vi "SimpleLiveAppProgrammableScanMode.vi"() -> ()   [LabVIEW 2020]
uses:
  C:/Users/Public/Documents/Photometrics/PMQI-LabViewSamples/Examples/2018/Dependencies/PVCamNET.dll
  Dependencies/PVCamNET.dll
panel:
  out "Exp. out":i32
  in  "Trigger Out Behaviour":string(combo)
  out "Boolean":bool
  in  "Scan Direction Reset":bool
  out "Scan Line Time":dbl format="%#_14g"
  in  "Scan Width":dbl
  in  "Scan Line Delay":dbl
  in  "Scan Direction":string(combo)
  in  "Scan Mode":string(combo)
  in  "Exposure Time":dbl
  in  "Live":bool
  in  "Camera Status":bool
  in  "Uninit":bool
  in  "Live stop":bool
  in  "Live start":bool
  in  "Open":bool
  # "SimpleLiveAppProgrammableScanMode.vi\n\nDescription:\nThis sample code lets the user use programmable scan\n mode in an event driven structure.\n\nSteps to run:\n1. Click \"Run\"\n2. Click \"Open\"\n3. Enter Exposure Time\n4. Select Scan Mode. \n5. Set Scan Line Delay or Scan Width\n6. Select Scan Direction\n7. Click \"Live start\"\n8. Click \"Live stop\"\n9. Click \"Close\""
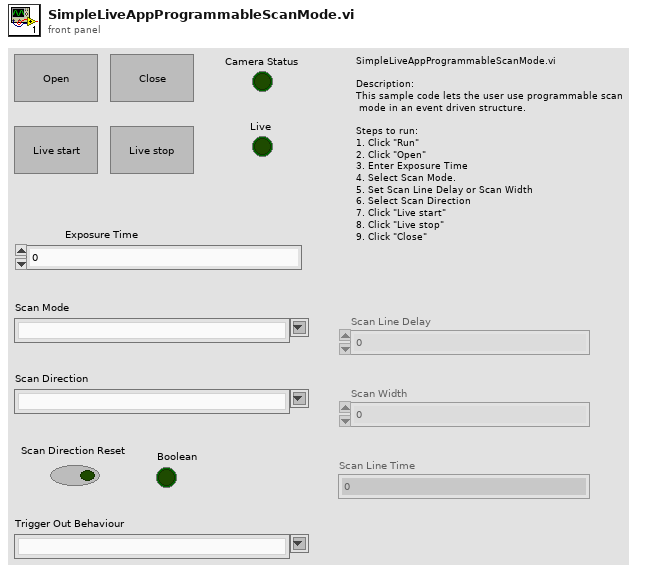
[diagram p1: front panel]
types:
  T1 = enum8{"Enabled", "Disabled", "Disabled and Grayed Out"}
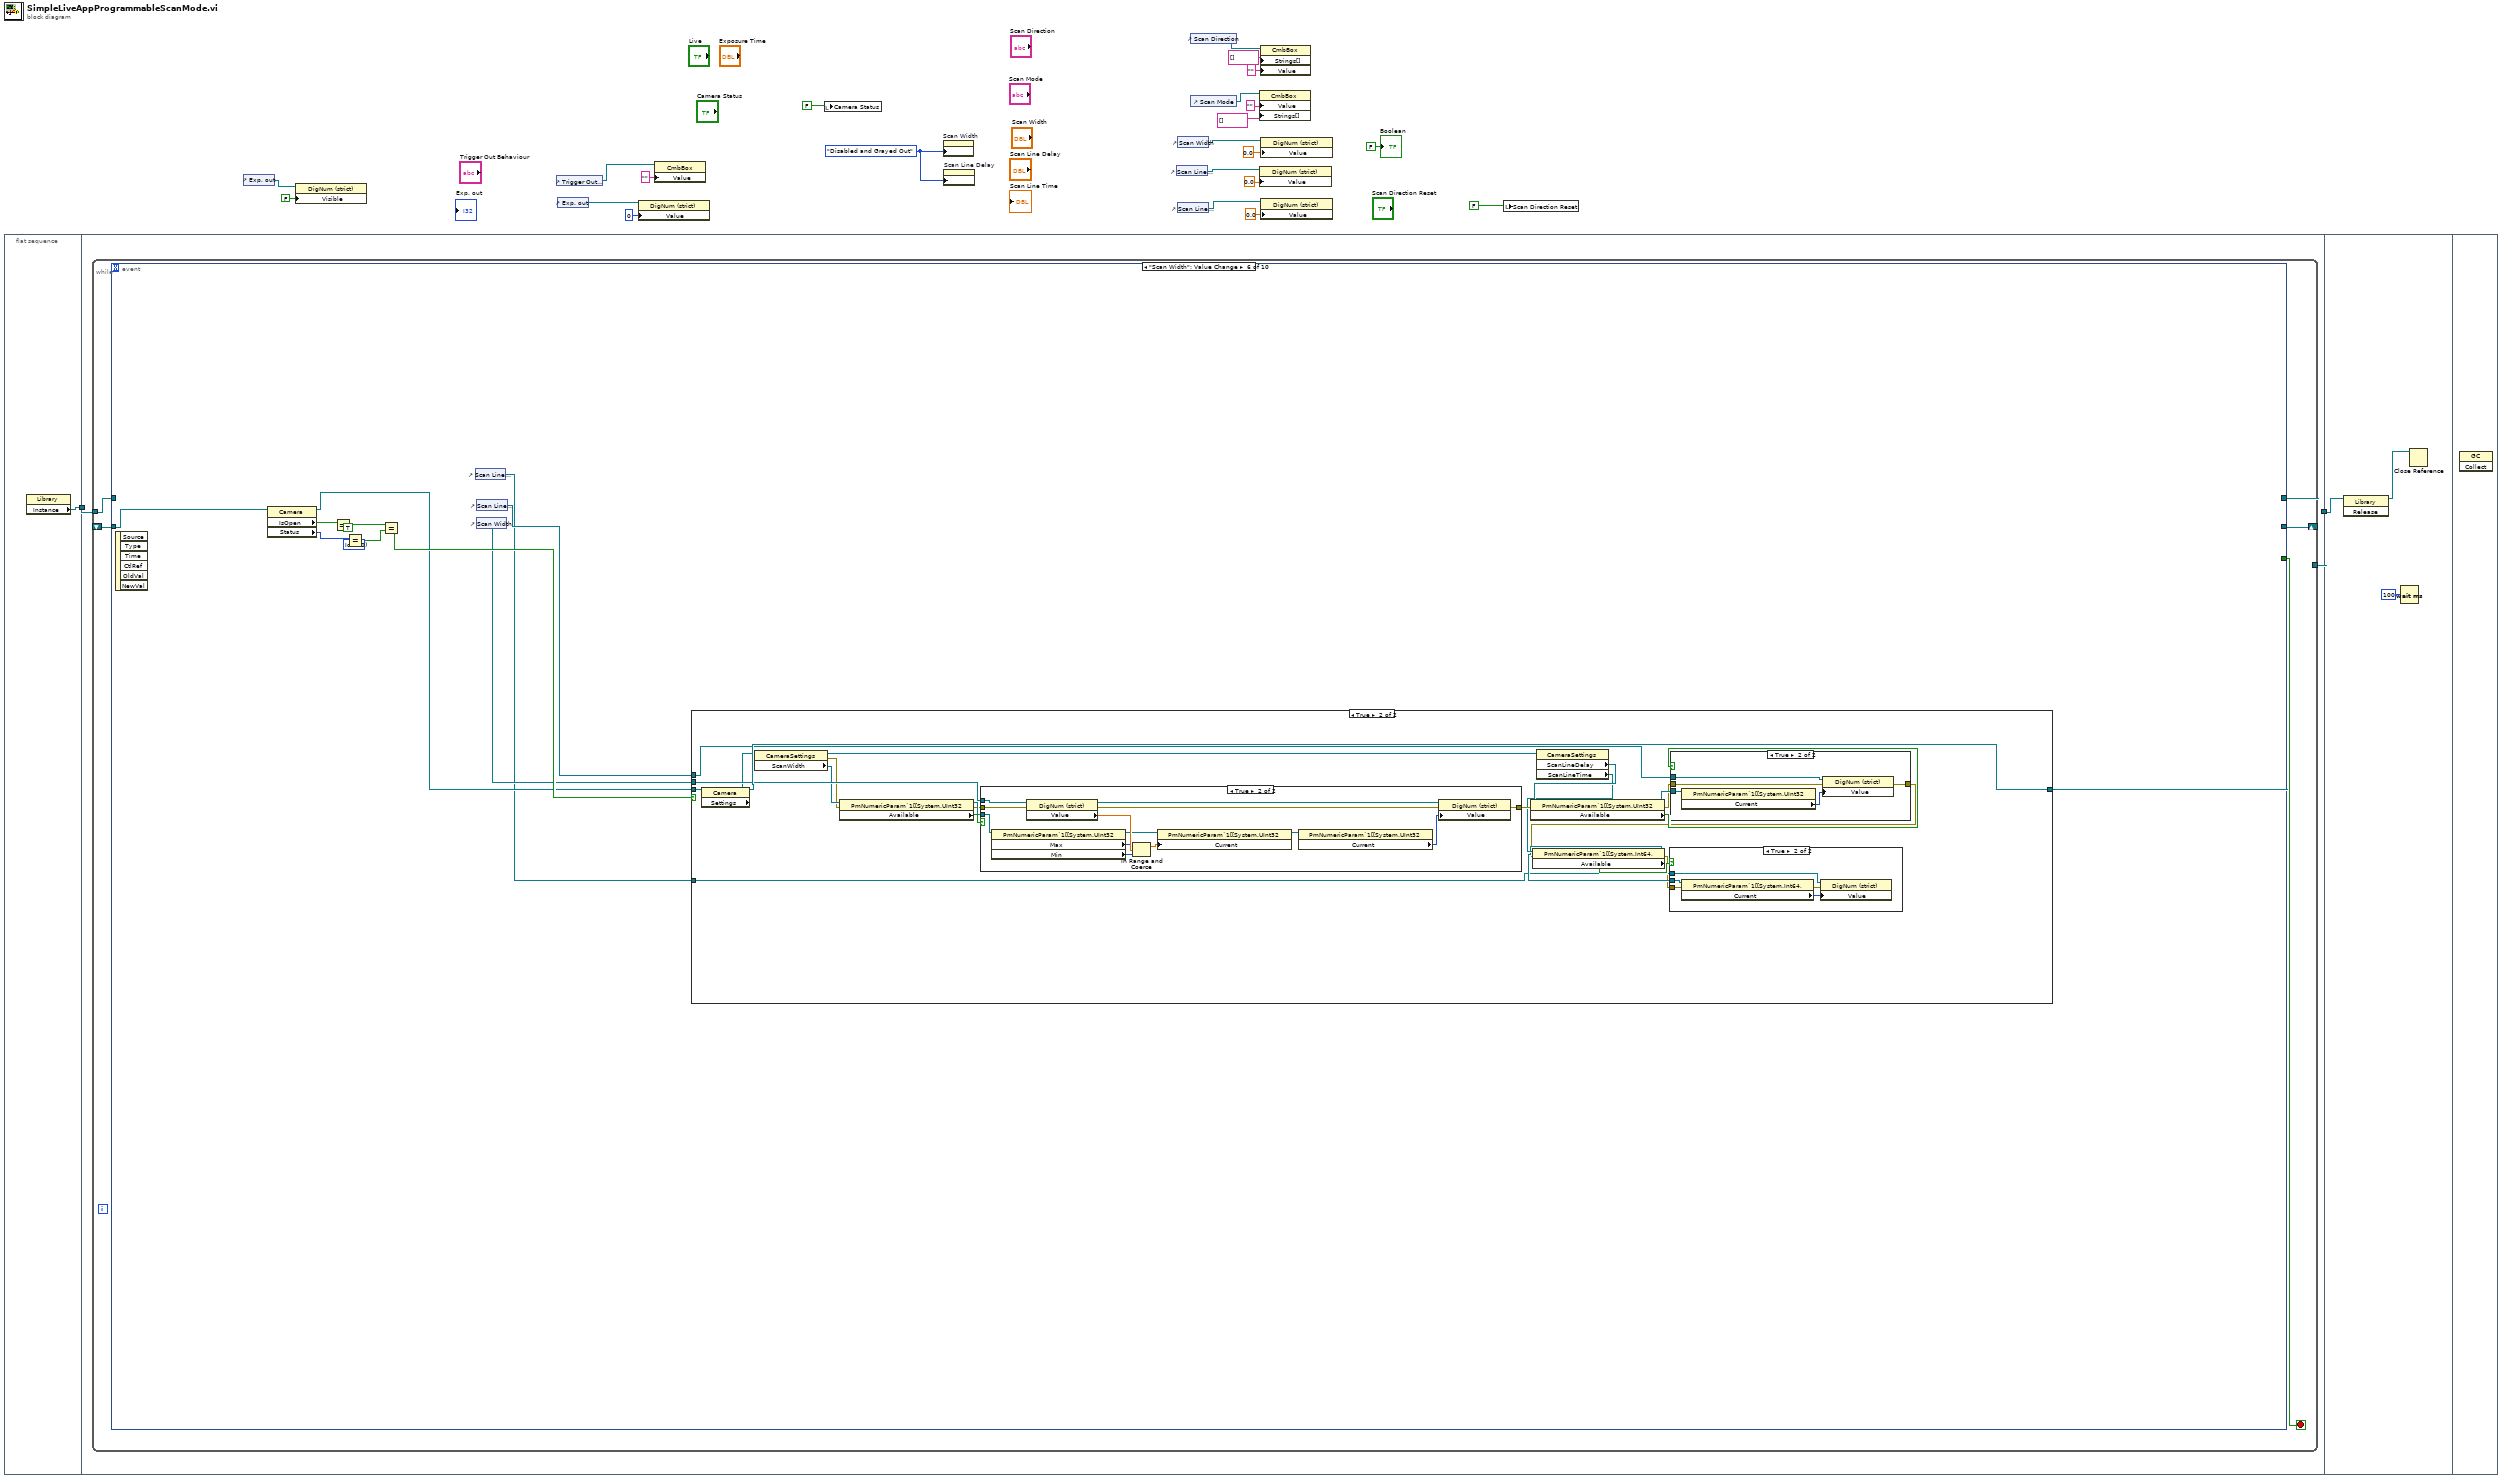
[diagram p0: block diagram]
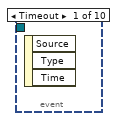
[diagram p2: hidden frame]
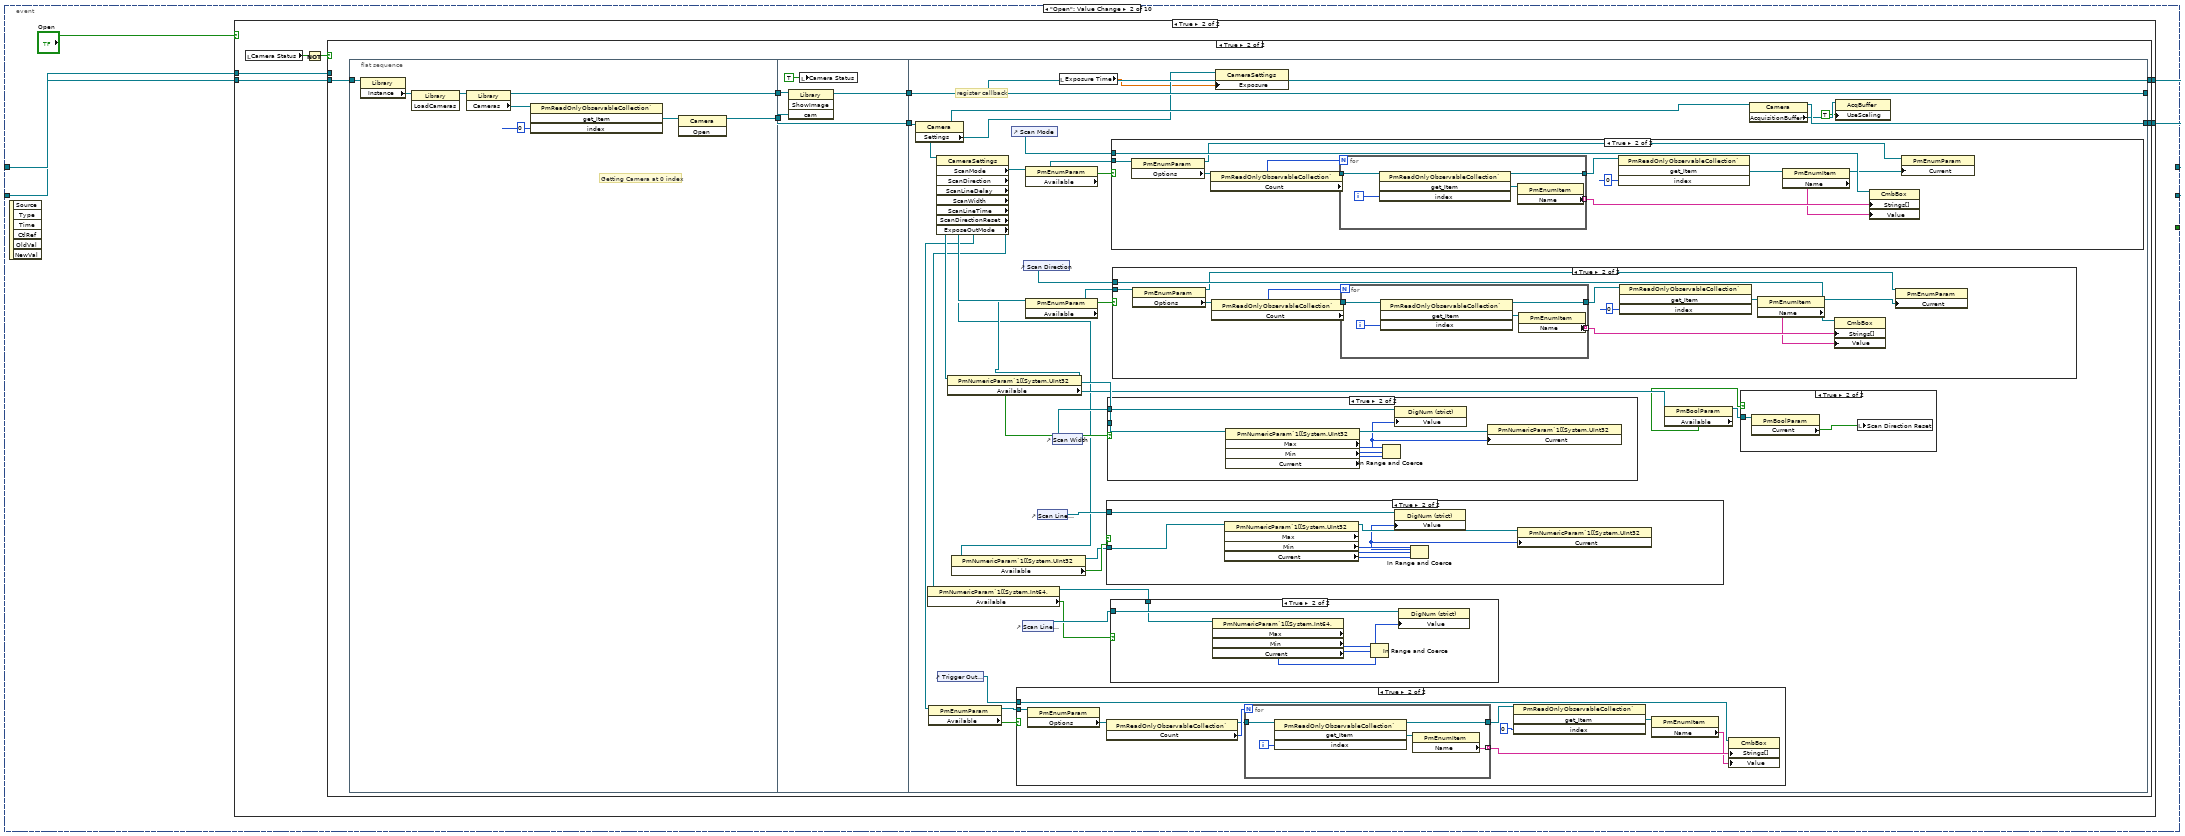
[diagram p3: hidden frame]
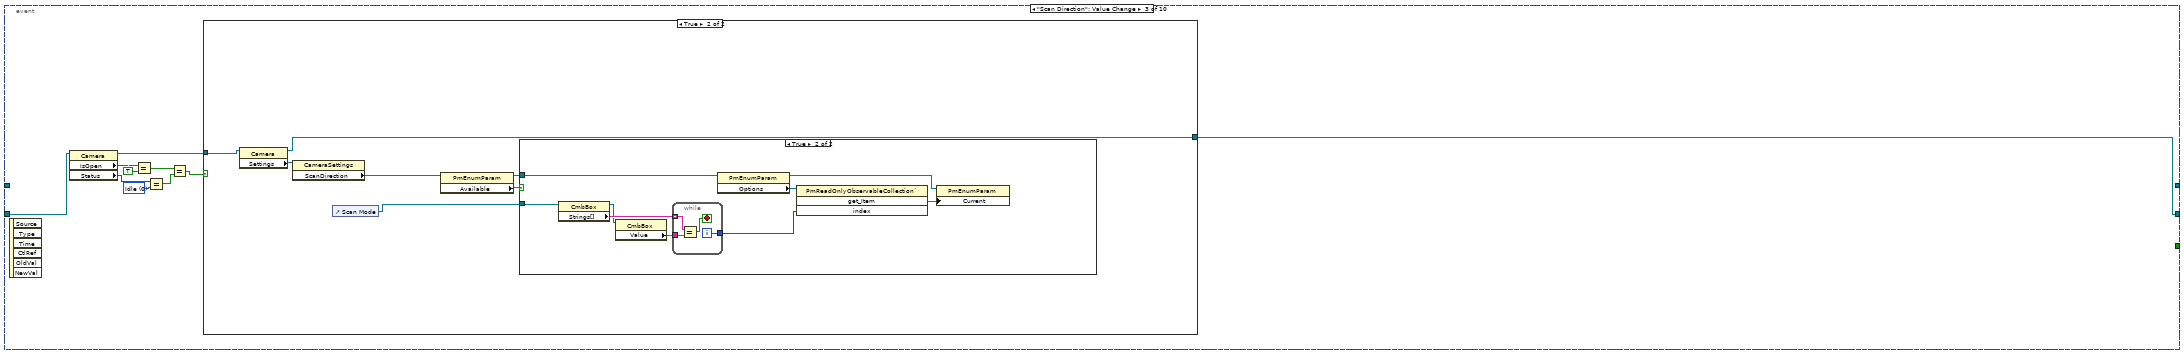
[diagram p13: hidden frame]
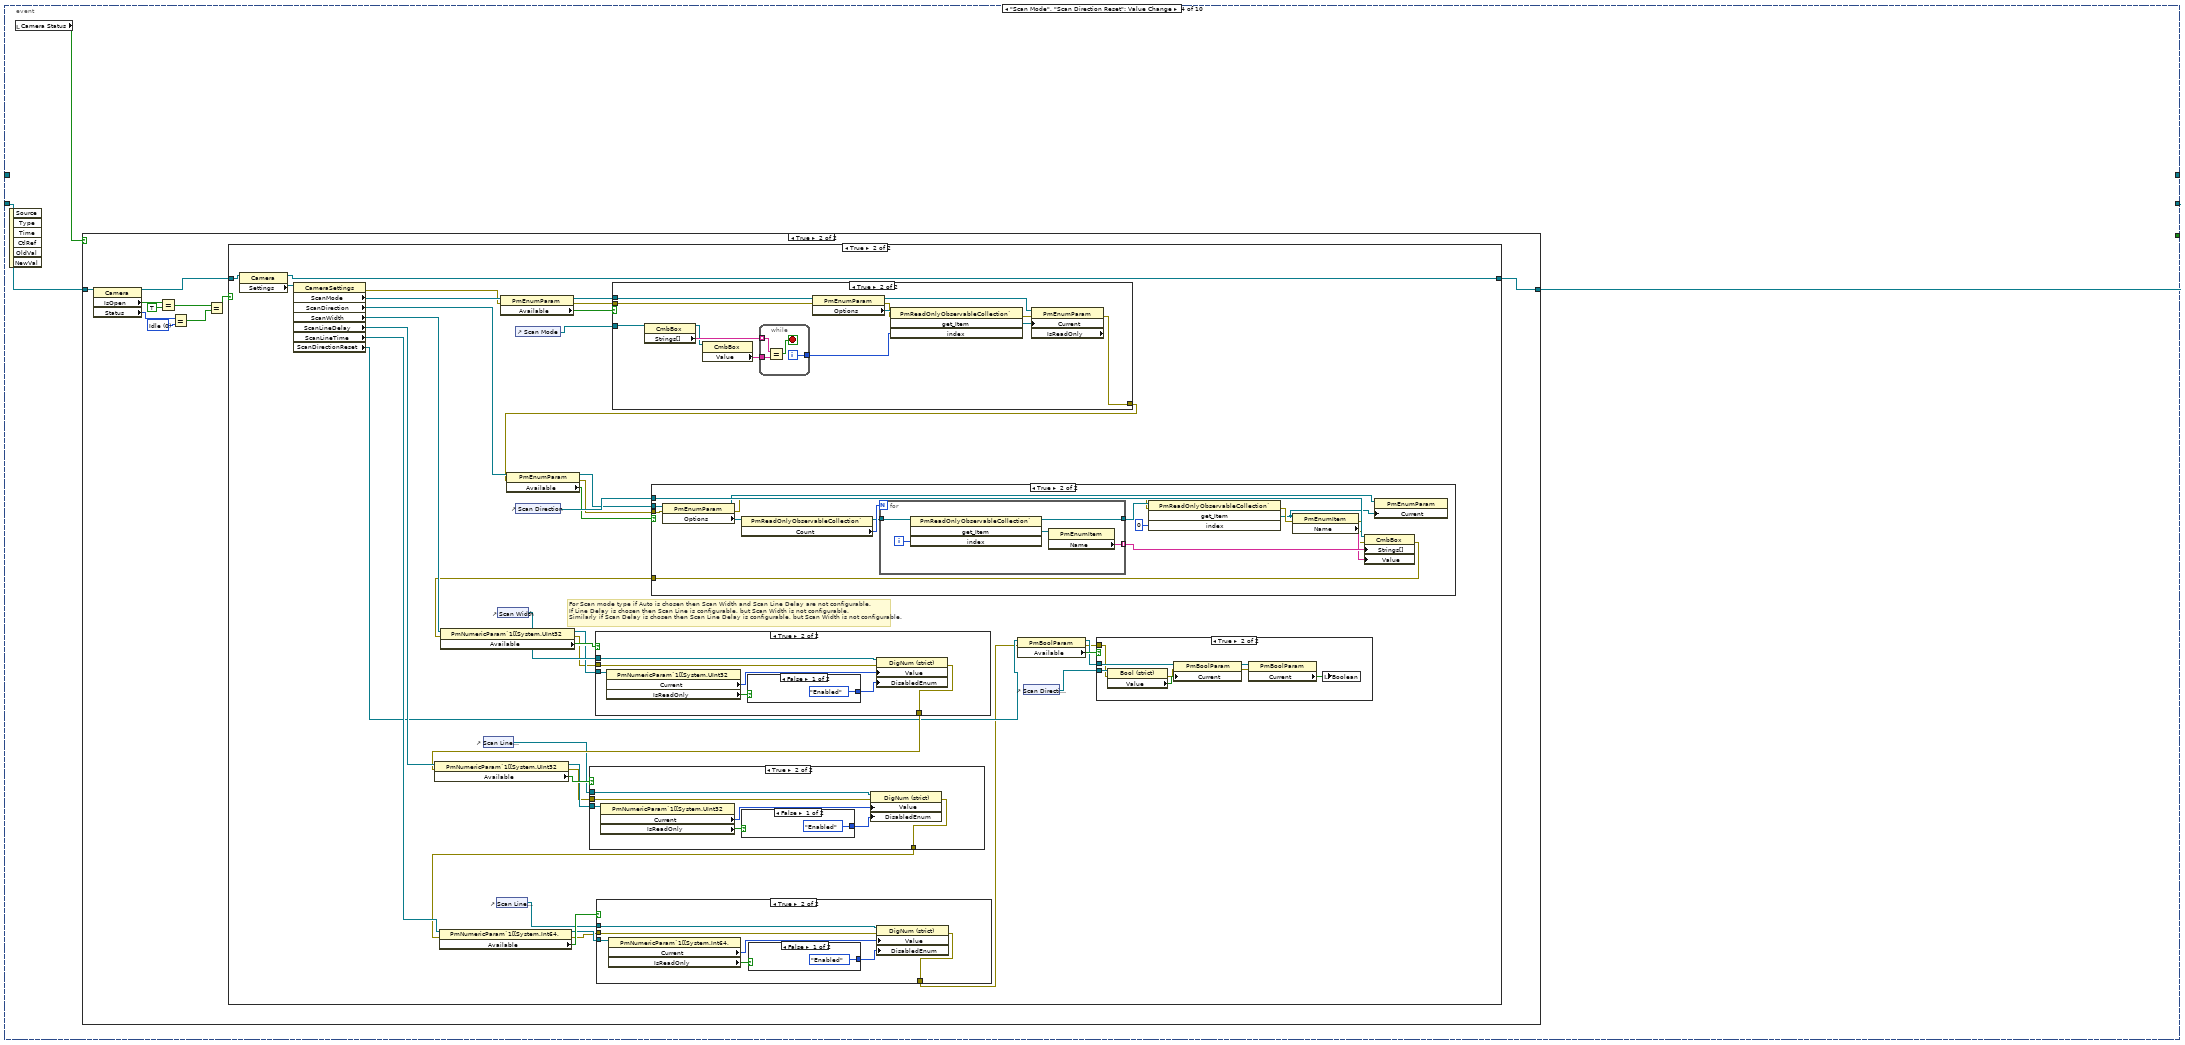
[diagram p16: hidden frame]
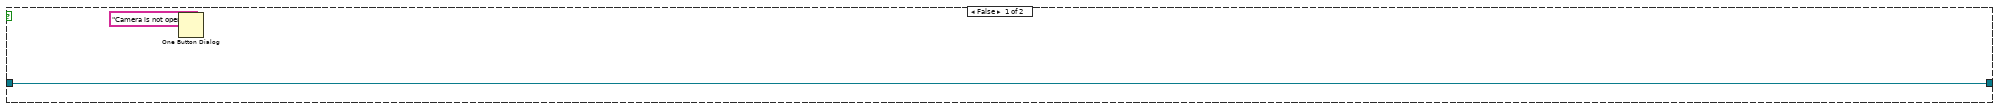
[diagram p17: hidden frame]
diagram:
  w9 = T1."Disabled and Grayed Out" ("Disabled")
  n1 = flat-sequence {
    tunnel: [w25] -> w24
    tunnel: w24 -> [w27]
    tunnel: [w26] -> w23
    tunnel: w23 -> [w591]
    frame #0 {
      n2 = property class="Library"() -> ("Instance"=w25:refnum<k24>)  [unwired: 2 in, 2 out]
    }
    frame #1 {
      n3 = while {
        tunnel: w27 -> [w32]
        shift-right: [w31] -> _
        shift-left: _ -> [w29]
        tunnel: [w30] -> w26
        stop <- w28 stop-if-true
        n4 = event shown="[5] \"Scan Width\": Value Change" {
          selector: _ -> [_ _ _ _ _ _ _ _ _ _]
          dyn-events: _ -> [_ _ _ _ _ _ _ _ _ _]
          timeout: _ -> [_ _ _ _ _ _ _ _ _ _]
          tunnel: w32 -> [_ w37 _ _ _ _ w460 w508 _ w563]
          tunnel: [_ w36 w173 w205 w337 w401 w461 w509 w538 w564] -> w31
          tunnel: [_ w35 _ _ _ _ w460 w508 _ w563] -> w30
          tunnel: w29 -> [_ w34 w177 w206 w343 w403 w462 w510 w539 w565]
          tunnel: [_ _ _ _ _ _ _ _ _ w562] -> w28
          event Timeout {
            n5 = event-data() -> ()  [unwired: 1 in, 3 out]
          }
          event "Open": Value Change {
            n6 = event-data() -> ()  [unwired: 1 in, 6 out]
            n7 = case shown="True" "Open" {
              tunnel: w37 -> [w39 w45]
              tunnel: [w38 w44] -> w36
              tunnel: [w39 w43] -> w35
              tunnel: w34 -> [w38 w40]
              frame False {
              }
              frame True {
                n8 = local read "Camera Status"() -> (w42:bool)
                n9 = Not(x=w42) -> (.not. x?=w41:bool)
                n10 = case shown="True" w41 {
                  tunnel: w45 -> [w46 w52]
                  tunnel: [w47 w51] -> w44
                  tunnel: [w46 w50] -> w43
                  tunnel: w40 -> [w47 _]
                  frame False {
                  }
                  frame True {
                    n11 = flat-sequence {
                      tunnel: w52 -> [w57]
                      tunnel: [w59] -> w54
                      tunnel: [w58] -> w53
                      tunnel: w54 -> [w65]
                      tunnel: w53 -> [w66]
                      tunnel: [w66] -> w49
                      tunnel: [w64] -> w48
                      tunnel: [w101] -> w50
                      tunnel: [w81] -> w51
                      tunnel: w49 -> [w100]
                      tunnel: w48 -> [w101]
                      frame #0 {
                        # "Getting Camera at 0 index"
                        n12 = property class="Library"(reference=w57) -> ("Instance"=w56:refnum<k24>)  [unwired: 1 in, 2 out]
                        n13 = invoke class="Library" method="LoadCameras"(reference=w56) -> (reference out=w55:refnum<k24>)  [unwired: 2 in, 2 out]
                        n14 = property class="Library"(reference=w55) -> (reference out=w59:refnum<k24>, "Cameras"=w62:refnum<k24>)  [unwired: 1 in, 1 out]
                        n15 = invoke class="PmReadOnlyObservableCollection`" method="get_Item"(reference=w62, "index"=0) -> ("get_Item"=w60:refnum<k24>)  [unwired: 2 in, 3 out]
                        n16 = invoke class="Camera" method="Open"(reference=w60) -> (reference out=w58:refnum<k24>)  [unwired: 2 in, 2 out]
                      }
                      frame #1 {
                        n17 = invoke class="Library" method="ShowImage"(reference=w65, "cam"=w66) -> (reference out=w64:refnum<k24>)  [unwired: 2 in, 3 out]
                        n18 = local write "Camera Status"(TRUE ("Camera Status")) -> ()
                      }
                      frame #2 {
                        # "register callback"
                        n19 = property class="Camera"(reference=w100) -> (reference out=w82:refnum<k24>, "Settings"=w71:refnum<k24>)  [unwired: 1 in, 1 out]
                        n20 = property class="CameraSettings"(reference=w71) -> ("ScanMode"=w99:refnum<k24>, "ScanDirection"=w95:refnum<k24>, "ScanLineDelay"=w90:refnum<k24>, "ScanWidth"=w77:refnum<k24>, "ScanLineTime"=w69:refnum<k24>, "ScanDirectionReset"=w85:refnum<k24>, "ExposeOutMode"=w73:refnum<k24>)  [unwired: 1 in, 2 out]
                        n21 = property class="PmNumericParam`1[[System.Int64,"(reference=w69) -> (reference out=w67:refnum<k24>, "Available"=w68:bool)  [unwired: 1 in, 1 out]
                        n22 = property class="PmEnumParam"(reference=w73) -> (reference out=w74:refnum<k24>, "Available"=w75:bool)  [unwired: 1 in, 1 out]
                        n23 = control-ref of="Trigger Out Behaviour"() -> (w72:refnum<vi>)
                        n24 = property class="PmNumericParam`1[[System.UInt32"(reference=w90) -> (reference out=w88:refnum<k24>, "Available"=w89:bool)  [unwired: 1 in, 1 out]
                        n25 = property class="PmNumericParam`1[[System.UInt32"(reference=w77) -> (reference out=w76:refnum<k24>, "Available"=w78:bool)  [unwired: 1 in, 1 out]
                        n26 = control-ref of="Scan Mode"() -> (w96:refnum<vi>)
                        n27 = case shown="True" w75 {
                          tunnel: w74 -> [_ w111]
                          tunnel: w72 -> [_ w102]
                          frame False {
                          }
                          frame True {
                            n28 = property class="PmEnumParam"(reference=w111) -> ("Options"=w110:refnum<k24>)  [unwired: 1 in, 2 out]
                            n29 = property class="PmReadOnlyObservableCollection`"(reference=w110) -> (reference out=w108:refnum<k24>, "Count"=w109:i32)  [unwired: 1 in, 1 out]
                            n30 = for {
                              N: w109 -> [_]
                              tunnel: w108 -> [w116]
                              tunnel: [w113] -> w105
                              tunnel: [w112] -> w104 mode=indexing
                              i -> [w115]
                              n31 = invoke class="PmReadOnlyObservableCollection`" method="get_Item"(reference=w116, "index"=w115) -> (reference out=w113:refnum<k24>, "get_Item"=w114:refnum<k24>)  [unwired: 2 in, 2 out]
                              n32 = property class="PmEnumItem"(reference=w114) -> ("Name"=w112:string)  [unwired: 1 in, 2 out]
                            }
                            n33 = invoke class="PmReadOnlyObservableCollection`" method="get_Item"(reference=w105, "index"=0) -> ("get_Item"=w106:refnum<k24>)  [unwired: 2 in, 3 out]
                            n34 = property class="PmEnumItem"(reference=w106) -> ("Name"=w103:string)  [unwired: 1 in, 2 out]
                            n35 = property class="CmbBox"(reference=w102, "Strings[]"=w104, "Value"=w103) -> ()  [unwired: 1 in, 2 out]
                          }
                        }
                        n36 = control-ref of="Scan Line Time"() -> (w86:refnum<vi>)
                        n37 = control-ref of="Scan Direction"() -> (w92:refnum<vi>)
                        n38 = property class="PmEnumParam"(reference=w99) -> (reference out=w97:refnum<k24>, "Available"=w98:bool)  [unwired: 1 in, 1 out]
                        n39 = property class="PmEnumParam"(reference=w95) -> (reference out=w93:refnum<k24>, "Available"=w94:bool)  [unwired: 1 in, 1 out]
                        n40 = control-ref of="Scan Line Delay"() -> (w87:refnum<vi>)
                        n41 = control-ref of="Scan Width"() -> (w91:refnum<vi>)
                        n42 = local read "Exposure Time"() -> (w70:dbl)
                        n43 = case shown="True" w78 {
                          tunnel: w87 -> [_ w128]
                          tunnel: w76 -> [_ w127]
                          frame False {
                          }
                          frame True {
                            n44 = property class="PmNumericParam`1[[System.UInt32"(reference=w127) -> (reference out=w126:refnum<k24>, "Max"=w129:u32, "Min"=w130:u32, "Current"=w131:u32)  [unwired: 1 in, 1 out]
                            n45 = In Range and Coerce(upper limit=w129, x=w131, lower limit=w130) -> (coerced(x)=w125:u32)  [unwired: 1 out]
                            n46 = property class="DigNum (strict)"(reference=w128, "Value"=w125) -> ()  [unwired: 1 in, 2 out]
                            n47 = property class="PmNumericParam`1[[System.UInt32"(reference=w126, "Current"=w125) -> ()  [unwired: 1 in, 2 out]
                          }
                        }
                        n48 = case shown="True" w89 {
                          tunnel: w91 -> [_ w135]
                          tunnel: w88 -> [_ w134]
                          frame False {
                          }
                          frame True {
                            n49 = property class="PmNumericParam`1[[System.UInt32"(reference=w134) -> (reference out=w133:refnum<k24>, "Max"=w136:u32, "Min"=w137:u32, "Current"=w138:u32)  [unwired: 1 in, 1 out]
                            n50 = In Range and Coerce(upper limit=w136, x=w138, lower limit=w137) -> (coerced(x)=w132:u32)  [unwired: 1 out]
                            n51 = property class="DigNum (strict)"(reference=w135, "Value"=w132) -> ()  [unwired: 1 in, 2 out]
                            n52 = property class="PmNumericParam`1[[System.UInt32"(reference=w133, "Current"=w132) -> ()  [unwired: 1 in, 2 out]
                          }
                        }
                        n53 = case shown="True" w68 {
                          tunnel: w86 -> [_ w120]
                          tunnel: w67 -> [_ w119]
                          frame False {
                          }
                          frame True {
                            n54 = property class="PmNumericParam`1[[System.Int64,"(reference=w119) -> ("Max"=w121:i64, "Min"=w122:i64, "Current"=w123:i64)  [unwired: 1 in, 2 out]
                            n55 = In Range and Coerce(upper limit=w121, x=w123, lower limit=w122) -> (coerced(x)=w124:i64)  [unwired: 1 out]
                            n56 = property class="DigNum (strict)"(reference=w120, "Value"=w124) -> ()  [unwired: 1 in, 2 out]
                          }
                        }
                        n57 = case shown="True" w98 {
                          tunnel: w97 -> [_ w167]
                          tunnel: w96 -> [_ w159]
                          frame False {
                          }
                          frame True {
                            n58 = property class="PmEnumParam"(reference=w167) -> (reference out=w158:refnum<k24>, "Options"=w166:refnum<k24>)  [unwired: 1 in, 1 out]
                            n59 = property class="PmReadOnlyObservableCollection`"(reference=w166) -> (reference out=w164:refnum<k24>, "Count"=w165:i32)  [unwired: 1 in, 1 out]
                            n60 = for {
                              N: w165 -> [_]
                              tunnel: w164 -> [w172]
                              tunnel: [w169] -> w162
                              tunnel: [w168] -> w161 mode=indexing
                              i -> [w171]
                              n61 = invoke class="PmReadOnlyObservableCollection`" method="get_Item"(reference=w172, "index"=w171) -> (reference out=w169:refnum<k24>, "get_Item"=w170:refnum<k24>)  [unwired: 2 in, 2 out]
                              n62 = property class="PmEnumItem"(reference=w170) -> ("Name"=w168:string)  [unwired: 1 in, 2 out]
                            }
                            n63 = invoke class="PmReadOnlyObservableCollection`" method="get_Item"(reference=w162, "index"=0) -> ("get_Item"=w157:refnum<k24>)  [unwired: 2 in, 3 out]
                            n64 = property class="PmEnumItem"(reference=w157) -> (reference out=w156:refnum<k24>, "Name"=w160:string)  [unwired: 1 in, 1 out]
                            n65 = property class="CmbBox"(reference=w159, "Strings[]"=w161, "Value"=w160) -> ()  [unwired: 1 in, 2 out]
                            n66 = property class="PmEnumParam"(reference=w158, "Current"=w156) -> ()  [unwired: 1 in, 2 out]
                          }
                        }
                        n67 = case shown="True" w94 {
                          tunnel: w93 -> [_ w150]
                          tunnel: w92 -> [_ w141]
                          frame False {
                          }
                          frame True {
                            n68 = property class="PmEnumParam"(reference=w150) -> (reference out=w140:refnum<k24>, "Options"=w149:refnum<k24>)  [unwired: 1 in, 1 out]
                            n69 = property class="PmReadOnlyObservableCollection`"(reference=w149) -> (reference out=w147:refnum<k24>, "Count"=w148:i32)  [unwired: 1 in, 1 out]
                            n70 = for {
                              N: w148 -> [_]
                              tunnel: w147 -> [w155]
                              tunnel: [w152] -> w144
                              tunnel: [w151] -> w143 mode=indexing
                              i -> [w154]
                              n71 = invoke class="PmReadOnlyObservableCollection`" method="get_Item"(reference=w155, "index"=w154) -> (reference out=w152:refnum<k24>, "get_Item"=w153:refnum<k24>)  [unwired: 2 in, 2 out]
                              n72 = property class="PmEnumItem"(reference=w153) -> ("Name"=w151:string)  [unwired: 1 in, 2 out]
                            }
                            n73 = invoke class="PmReadOnlyObservableCollection`" method="get_Item"(reference=w144, "index"=0) -> ("get_Item"=w145:refnum<k24>)  [unwired: 2 in, 3 out]
                            n74 = property class="PmEnumItem"(reference=w145) -> (reference out=w139:refnum<k24>, "Name"=w142:string)  [unwired: 1 in, 1 out]
                            n75 = property class="CmbBox"(reference=w141, "Strings[]"=w143, "Value"=w142) -> ()  [unwired: 1 in, 2 out]
                            n76 = property class="PmEnumParam"(reference=w140, "Current"=w139) -> ()  [unwired: 1 in, 2 out]
                          }
                        }
                        n77 = property class="CameraSettings"(reference=w71, "Exposure"=w70) -> ()  [unwired: 1 in, 2 out]
                        n78 = property class="PmBoolParam"(reference=w85) -> (reference out=w83:refnum<k24>, "Available"=w84:bool)  [unwired: 1 in, 1 out]
                        n79 = case shown="True" w84 {
                          tunnel: w83 -> [_ w118]
                          frame False {
                          }
                          frame True {
                            n80 = property class="PmBoolParam"(reference=w118) -> ("Current"=w117:bool)  [unwired: 1 in, 2 out]
                            n81 = local write "Scan Direction Reset"(w117) -> ()
                          }
                        }
                        n82 = property class="Camera"(reference=w82) -> (reference out=w81:refnum<k24>, "AcquisitionBuffer"=w80:refnum<k24>)  [unwired: 1 in, 1 out]
                        n83 = property class="AcqBuffer"(reference=w80, "UseScaling"=TRUE) -> ()  [unwired: 1 in, 2 out]
                      }
                    }
                  }
                }
              }
            }
          }
          event "Scan Direction": Value Change {
            w181 = 0 items=["Idle", "Capturing"] ("Status")
            n84 = event-data() -> ()  [unwired: 1 in, 6 out]
            n85 = property class="Camera"(reference=w177) -> (reference out=w174:refnum<k24>, "IsOpen"=w180:bool, "Status"=w182:i32)  [unwired: 1 in, 1 out]
            n86 = Equal?(x=w180, y=TRUE) -> (x = y?=w176:bool)
            n87 = Equal?(x=w182, y=w181) -> (x = y?=w178:bool)
            n88 = Equal?(x=w176, y=w178) -> (x = y?=w175:bool)
            n89 = case shown="True" w175 {
              tunnel: w174 -> [w183 w187]
              tunnel: [w183 w184] -> w173
              frame False {
              }
              frame True {
                n90 = property class="Camera"(reference=w187) -> (reference out=w184:refnum<k24>, "Settings"=w188:refnum<k24>)  [unwired: 1 in, 1 out]
                n91 = property class="CameraSettings"(reference=w188) -> ("ScanDirection"=w186:refnum<k24>)  [unwired: 1 in, 2 out]
                n92 = control-ref of="Scan Mode"() -> (w185:refnum<vi>)
                n93 = property class="PmEnumParam"(reference=w186) -> (reference out=w189:refnum<k24>, "Available"=w190:bool)  [unwired: 1 in, 1 out]
                n94 = case shown="True" w190 {
                  tunnel: w189 -> [_ w198]
                  tunnel: w185 -> [_ w191]
                  frame False {
                  }
                  frame True {
                    n95 = property class="CmbBox"(reference=w191) -> (reference out=w193:refnum<vi>, "Strings[]"=w199:string[])  [unwired: 1 in, 1 out]
                    n96 = property class="CmbBox"(reference=w193) -> ("Value"=w192:string)  [unwired: 1 in, 2 out]
                    n97 = while {
                      tunnel: w199 -> [w203] mode=indexing
                      tunnel: [w201] -> w196
                      tunnel: w192 -> [w200]
                      i -> [w201]
                      stop <- w202 stop-if-true
                      n98 = Equal?(x=w203, y=w200) -> (x = y?=w202:bool)
                    }
                    n99 = property class="PmEnumParam"(reference=w198) -> (reference out=w195:refnum<k24>, "Options"=w197:refnum<k24>)  [unwired: 1 in, 1 out]
                    n100 = invoke class="PmReadOnlyObservableCollection`" method="get_Item"(reference=w197, "index"=w196) -> ("get_Item"=w194:refnum<k24>)  [unwired: 2 in, 3 out]
                    n101 = property class="PmEnumParam"(reference=w195, "Current"=w194) -> ()  [unwired: 1 in, 2 out]
                  }
                }
              }
            }
          }
          event "Scan Mode", "Scan Direction Reset": Value Change {
            n102 = event-data() -> ()  [unwired: 1 in, 6 out]
            n103 = local read "Camera Status"() -> (w204:bool)
            n104 = case shown="True" w204 {
              tunnel: w206 -> [w207 w212]
              tunnel: [w207 w210] -> w205
              frame False {
                n105 = One Button Dialog(message="Camera is not open") -> ()  [unwired: 1 in, 1 out]
              }
              frame True {
                w217 = 0 items=["Idle", "Capturing"] ("Status")
                n106 = property class="Camera"(reference=w212) -> (reference out=w211:refnum<k24>, "IsOpen"=w216:bool, "Status"=w218:i32)  [unwired: 1 in, 1 out]
                n107 = Equal?(x=w216, y=TRUE) -> (x = y?=w214:bool)
                n108 = Equal?(x=w218, y=w217) -> (x = y?=w213:bool)
                n109 = Equal?(x=w214, y=w213) -> (x = y?=w209:bool)
                n110 = case shown="True" w209 {
                  tunnel: w211 -> [w219 w258]
                  tunnel: [w219 w253] -> w210
                  frame False {
                  }
                  frame True {
                    # "For Scan mode type if Auto is chosen then Scan Width and Scan Line Delay are not configurable.\nIf Line Delay is chosen then Scan Line is configurable, but Scan Width is not configurable.\nSimilarly if Scan Delay is chosen then Scan Line Delay is configurable, but Scan Width is not configurable."
                    n111 = property class="Camera"(reference=w258) -> (reference out=w253:refnum<k24>, "Settings"=w257:refnum<k24>)  [unwired: 1 in, 1 out]
                    n112 = property class="CameraSettings"(reference=w257) -> (error out=w250:errorcluster, "ScanMode"=w256:refnum<k24>, "ScanDirection"=w252:refnum<k24>, "ScanWidth"=w248:refnum<k24>, "ScanLineDelay"=w247:refnum<k24>, "ScanLineTime"=w236:refnum<k24>, "ScanDirectionReset"=w225:refnum<k24>)  [unwired: 1 in, 1 out]
                    n113 = control-ref of="Scan Line Delay"() -> (w227:refnum<vi>)
                    n114 = control-ref of="Scan Line Time"() -> (w230:refnum<vi>)
                    n115 = control-ref of="Scan Width"() -> (w243:refnum<vi>)
                    n116 = property class="PmEnumParam"(reference=w256, error in=w250) -> (reference out=w254:refnum<k24>, error out=w251:errorcluster, "Available"=w255:bool)
                    n117 = control-ref of="Scan Mode"() -> (w249:refnum<vi>)
                    n118 = control-ref of="Scan Direction"() -> (w246:refnum<vi>)
                    n119 = case shown="True" w255 {
                      tunnel: w254 -> [_ w331]
                      tunnel: w249 -> [_ w326]
                      tunnel: w251 -> [w319 w325]
                      tunnel: [w319 w320] -> w235
                      frame False {
                      }
                      frame True {
                        n120 = property class="CmbBox"(reference=w326) -> (reference out=w327:refnum<vi>, "Strings[]"=w332:string[])  [unwired: 1 in, 1 out]
                        n121 = property class="CmbBox"(reference=w327) -> ("Value"=w322:string)  [unwired: 1 in, 2 out]
                        n122 = while {
                          tunnel: w332 -> [w336] mode=indexing
                          tunnel: [w334] -> w329
                          tunnel: w322 -> [w333]
                          i -> [w334]
                          stop <- w335 stop-if-true
                          n123 = Equal?(x=w336, y=w333) -> (x = y?=w335:bool)
                        }
                        n124 = property class="PmEnumParam"(reference=w331, error in=w325) -> (reference out=w328:refnum<k24>, error out=w324:errorcluster, "Options"=w330:refnum<k24>)
                        n125 = invoke class="PmReadOnlyObservableCollection`" method="get_Item"(reference=w330, error in=w324, "index"=w329) -> (error out=w323:errorcluster, "get_Item"=w321:refnum<k24>)  [unwired: 1 in, 2 out]
                        n126 = property class="PmEnumParam" props=["Current", "IsReadOnly"](reference=w328, error in=w323, "Current"=w321) -> (error out=w320:errorcluster)  [unwired: 2 out]
                      }
                    }
                    n127 = property class="PmEnumParam"(reference=w252, error in=w235) -> (reference out=w244:refnum<k24>, error out=w238:errorcluster, "Available"=w245:bool)
                    n128 = case shown="True" w245 {
                      tunnel: w244 -> [_ w313]
                      tunnel: w246 -> [_ w305]
                      tunnel: w238 -> [w297 w304]
                      tunnel: [w297 w298] -> w237
                      frame False {
                      }
                      frame True {
                        n129 = property class="PmEnumParam"(reference=w313, error in=w304) -> (reference out=w299:refnum<k24>, error out=w303:errorcluster, "Options"=w312:refnum<k24>)
                        n130 = property class="PmReadOnlyObservableCollection`"(reference=w312) -> (reference out=w310:refnum<k24>, "Count"=w311:i32)  [unwired: 1 in, 1 out]
                        n131 = for {
                          N: w311 -> [_]
                          tunnel: w310 -> [w318]
                          tunnel: [w315] -> w308
                          tunnel: [w314] -> w307 mode=indexing
                          i -> [w317]
                          n132 = invoke class="PmReadOnlyObservableCollection`" method="get_Item"(reference=w318, "index"=w317) -> (reference out=w315:refnum<k24>, "get_Item"=w316:refnum<k24>)  [unwired: 2 in, 2 out]
                          n133 = property class="PmEnumItem"(reference=w316) -> ("Name"=w314:string)  [unwired: 1 in, 2 out]
                        }
                        n134 = invoke class="PmReadOnlyObservableCollection`" method="get_Item"(reference=w308, error in=w303, "index"=0) -> (error out=w302:errorcluster, "get_Item"=w300:refnum<k24>)  [unwired: 1 in, 2 out]
                        n135 = property class="PmEnumItem"(reference=w300, error in=w302) -> (error out=w301:errorcluster, "Name"=w306:string)  [unwired: 1 out]
                        n136 = property class="CmbBox"(reference=w305, error in=w301, "Strings[]"=w307, "Value"=w306) -> (error out=w298:errorcluster)  [unwired: 1 out]
                        n137 = property class="PmEnumParam"(reference=w299, "Current"=w300) -> ()  [unwired: 1 in, 2 out]
                      }
                    }
                    n138 = property class="PmNumericParam`1[[System.UInt32"(reference=w248, error in=w237) -> (reference out=w241:refnum<k24>, error out=w240:errorcluster, "Available"=w242:bool)
                    n139 = case shown="True" w242 {
                      tunnel: w243 -> [_ w293]
                      tunnel: w241 -> [_ w290]
                      tunnel: w240 -> [w287 w292]
                      tunnel: [w287 w291] -> w239
                      frame False {
                      }
                      frame True {
                        n140 = property class="PmNumericParam`1[[System.UInt32"(reference=w290) -> ("Current"=w294:u32, "IsReadOnly"=w289:bool)  [unwired: 1 in, 2 out]
                        n141 = case shown="False" w289 {
                          tunnel: [T1."Enabled" ("Disabled") T1."Disabled and Grayed Out" ("Disabled")] -> w288
                          frame False {
                          }
                          frame True {
                          }
                        }
                        n142 = property class="DigNum (strict)"(reference=w293, error in=w292, "Value"=w294, "DisabledEnum"=w288) -> (error out=w291:errorcluster)  [unwired: 1 out]
                      }
                    }
                    n143 = property class="PmNumericParam`1[[System.UInt32"(reference=w247, error in=w239) -> (reference out=w232:refnum<k24>, error out=w226:errorcluster, "Available"=w233:bool)
                    n144 = case shown="True" w233 {
                      tunnel: w227 -> [_ w283]
                      tunnel: w232 -> [_ w280]
                      tunnel: w226 -> [w277 w282]
                      tunnel: [w277 w281] -> w229
                      frame False {
                      }
                      frame True {
                        n145 = property class="PmNumericParam`1[[System.UInt32"(reference=w280) -> ("Current"=w284:u32, "IsReadOnly"=w279:bool)  [unwired: 1 in, 2 out]
                        n146 = case shown="False" w279 {
                          tunnel: [T1."Enabled" ("Disabled") T1."Disabled and Grayed Out" ("Disabled")] -> w278
                          frame False {
                          }
                          frame True {
                          }
                        }
                        n147 = property class="DigNum (strict)"(reference=w283, error in=w282, "Value"=w284, "DisabledEnum"=w278) -> (error out=w281:errorcluster)  [unwired: 1 out]
                      }
                    }
                    n148 = property class="PmNumericParam`1[[System.Int64,"(reference=w236, error in=w229) -> (reference out=w231:refnum<k24>, error out=w228:errorcluster, "Available"=w234:bool)
                    n149 = case shown="True" w234 {
                      tunnel: w230 -> [_ w273]
                      tunnel: w231 -> [_ w270]
                      tunnel: w228 -> [w267 w272]
                      tunnel: [w267 w271] -> w221
                      frame False {
                      }
                      frame True {
                        n150 = property class="PmNumericParam`1[[System.Int64,"(reference=w270) -> ("Current"=w274:i64, "IsReadOnly"=w269:bool)  [unwired: 1 in, 2 out]
                        n151 = case shown="False" w269 {
                          tunnel: [T1."Enabled" ("Disabled") T1."Disabled and Grayed Out" ("Disabled")] -> w268
                          frame False {
                          }
                          frame True {
                          }
                        }
                        n152 = property class="DigNum (strict)"(reference=w273, error in=w272, "Value"=w274, "DisabledEnum"=w268) -> (error out=w271:errorcluster)  [unwired: 1 out]
                      }
                    }
                    n153 = property class="PmBoolParam"(reference=w225, error in=w221) -> (reference out=w223:refnum<k24>, error out=w220:errorcluster, "Available"=w224:bool)
                    n154 = control-ref of="Scan Direction Reset"() -> (w222:refnum<vi>)
                    n155 = case shown="True" w224 {
                      tunnel: w223 -> [_ w264]
                      tunnel: w222 -> [_ w266]
                      tunnel: w220 -> [_ w261]
                      frame False {
                      }
                      frame True {
                        n156 = property class="Bool (strict)"(reference=w266, error in=w261) -> (error out=w260:errorcluster, "Value"=w265:bool)  [unwired: 1 out]
                        n157 = property class="PmBoolParam"(reference=w264, error in=w260, "Current"=w265) -> (reference out=w263:refnum<k24>, error out=w259:errorcluster)
                        n158 = property class="PmBoolParam"(reference=w263, error in=w259) -> ("Current"=w262:bool)  [unwired: 2 out]
                        n159 = local write "Boolean"(w262) -> ()
                      }
                    }
                  }
                }
              }
            }
          }
          event "Scan Line Delay": Value Change {
            w348 = 0 items=["Idle", "Capturing"] ("Status")
            n160 = event-data() -> ()  [unwired: 1 in, 6 out]
            n161 = property class="Camera"(reference=w343) -> (reference out=w342:refnum<k24>, "IsOpen"=w347:bool, "Status"=w349:i32)  [unwired: 1 in, 1 out]
            n162 = Equal?(x=w347, y=TRUE) -> (x = y?=w345:bool)
            n163 = Equal?(x=w349, y=w348) -> (x = y?=w344:bool)
            n164 = Equal?(x=w345, y=w344) -> (x = y?=w341:bool)
            n165 = control-ref of="Scan Line Time"() -> (w338:refnum<vi>)
            n166 = control-ref of="Scan Line Delay"() -> (w339:refnum<vi>)
            n167 = control-ref of="Scan Width"() -> (w340:refnum<vi>)
            n168 = case shown="True" w341 {
              tunnel: w342 -> [w350 w372]
              tunnel: [w350 w371] -> w337
              tunnel: w339 -> [_ w370]
              tunnel: w340 -> [_ w369]
              tunnel: w338 -> [_ w353]
              frame False {
              }
              frame True {
                n169 = property class="Camera"(reference=w372) -> (reference out=w371:refnum<k24>, "Settings"=w368:refnum<k24>)  [unwired: 1 in, 1 out]
                n170 = property class="CameraSettings"(reference=w368) -> (reference out=w358:refnum<k24>, error out=w364:errorcluster, "ScanLineDelay"=w367:refnum<k24>)  [unwired: 1 in]
                n171 = property class="PmNumericParam`1[[System.UInt32"(reference=w367, error in=w364) -> (reference out=w365:refnum<k24>, error out=w363:errorcluster, "Available"=w366:bool)
                n172 = case shown="True" w366 {
                  tunnel: w370 -> [_ w389]
                  tunnel: w365 -> [_ w388]
                  tunnel: w363 -> [w384 w387]
                  tunnel: [w384 w385] -> w359
                  frame False {
                  }
                  frame True {
                    n173 = property class="PmNumericParam`1[[System.UInt32"(reference=w388) -> (reference out=w392:refnum<k24>, "Max"=w390:u32, "Min"=w391:u32)  [unwired: 1 in, 1 out]
                    n174 = property class="DigNum (strict)"(reference=w389, error in=w387) -> (reference out=w396:refnum<vi>, error out=w386:errorcluster, "Value"=w395:dbl)
                    n175 = In Range and Coerce(upper limit=w390, x=w395, lower limit=w391) -> (coerced(x)=w394:dbl)  [unwired: 1 out]
                    n176 = property class="PmNumericParam`1[[System.UInt32"(reference=w392, "Current"=w394) -> (reference out=w393:refnum<k24>)  [unwired: 1 in, 1 out]
                    n177 = property class="PmNumericParam`1[[System.UInt32"(reference=w393) -> ("Current"=w397:u32)  [unwired: 1 in, 2 out]
                    n178 = property class="DigNum (strict)"(reference=w396, error in=w386, "Value"=w397) -> (error out=w385:errorcluster)  [unwired: 1 out]
                  }
                }
                n179 = property class="CameraSettings"(reference=w358) -> ("ScanWidth"=w357:refnum<k24>, "ScanLineTime"=w356:refnum<k24>)  [unwired: 1 in, 2 out]
                n180 = property class="PmNumericParam`1[[System.UInt32"(reference=w357, error in=w359) -> (reference out=w361:refnum<k24>, error out=w360:errorcluster, "Available"=w362:bool)
                n181 = case shown="True" w362 {
                  tunnel: w369 -> [_ w380]
                  tunnel: w361 -> [_ w383]
                  tunnel: w360 -> [w378 w381]
                  tunnel: [w378 w382] -> w352
                  frame False {
                  }
                  frame True {
                    n182 = property class="PmNumericParam`1[[System.UInt32"(reference=w383) -> ("Current"=w379:u32)  [unwired: 1 in, 2 out]
                    n183 = property class="DigNum (strict)"(reference=w380, error in=w381, "Value"=w379) -> (error out=w382:errorcluster)  [unwired: 1 out]
                  }
                }
                n184 = property class="PmNumericParam`1[[System.Int64,"(reference=w356, error in=w352) -> (reference out=w354:refnum<k24>, error out=w351:errorcluster, "Available"=w355:bool)
                n185 = case shown="True" w355 {
                  tunnel: w354 -> [_ w377]
                  tunnel: w353 -> [_ w375]
                  tunnel: w351 -> [_ w374]
                  frame False {
                  }
                  frame True {
                    n186 = property class="PmNumericParam`1[[System.Int64,"(reference=w377, error in=w374) -> (error out=w373:errorcluster, "Current"=w376:i64)  [unwired: 1 out]
                    n187 = property class="DigNum (strict)"(reference=w375, error in=w373, "Value"=w376) -> ()  [unwired: 2 out]
                  }
                }
              }
            }
          }
          event "Scan Width": Value Change {
            w409 = 0 items=["Idle", "Capturing"] ("Status")
            n188 = event-data() -> ()  [unwired: 1 in, 6 out]
            n189 = property class="Camera"(reference=w403) -> (reference out=w402:refnum<k24>, "IsOpen"=w408:bool, "Status"=w410:i32)  [unwired: 1 in, 1 out]
            n190 = Equal?(x=w408, y=TRUE) -> (x = y?=w406:bool)
            n191 = Equal?(x=w410, y=w409) -> (x = y?=w405:bool)
            n192 = Equal?(x=w406, y=w405) -> (x = y?=w404:bool)
            n193 = control-ref of="Scan Line Time"() -> (w398:refnum<vi>)
            n194 = control-ref of="Scan Width"() -> (w400:refnum<vi>)
            n195 = control-ref of="Scan Line Delay"() -> (w399:refnum<vi>)
            n196 = case shown="True" w404 {
              tunnel: w402 -> [w411 w433]
              tunnel: [w411 w432] -> w401
              tunnel: w400 -> [_ w431]
              tunnel: w399 -> [_ w430]
              tunnel: w398 -> [_ w415]
              frame False {
              }
              frame True {
                n197 = property class="Camera"(reference=w433) -> (reference out=w432:refnum<k24>, "Settings"=w429:refnum<k24>)  [unwired: 1 in, 1 out]
                n198 = property class="CameraSettings"(reference=w429) -> (reference out=w412:refnum<k24>, error out=w425:errorcluster, "ScanWidth"=w428:refnum<k24>)  [unwired: 1 in]
                n199 = property class="PmNumericParam`1[[System.UInt32"(reference=w428, error in=w425) -> (reference out=w426:refnum<k24>, error out=w424:errorcluster, "Available"=w427:bool)
                n200 = case shown="True" w427 {
                  tunnel: w431 -> [_ w450]
                  tunnel: w426 -> [_ w449]
                  tunnel: w424 -> [w445 w448]
                  tunnel: [w445 w446] -> w420
                  frame False {
                  }
                  frame True {
                    n201 = property class="PmNumericParam`1[[System.UInt32"(reference=w449) -> (reference out=w453:refnum<k24>, "Max"=w451:u32, "Min"=w452:u32)  [unwired: 1 in, 1 out]
                    n202 = property class="DigNum (strict)"(reference=w450, error in=w448) -> (reference out=w457:refnum<vi>, error out=w447:errorcluster, "Value"=w456:dbl)
                    n203 = In Range and Coerce(upper limit=w451, x=w456, lower limit=w452) -> (coerced(x)=w455:dbl)  [unwired: 1 out]
                    n204 = property class="PmNumericParam`1[[System.UInt32"(reference=w453, "Current"=w455) -> (reference out=w454:refnum<k24>)  [unwired: 1 in, 1 out]
                    n205 = property class="PmNumericParam`1[[System.UInt32"(reference=w454) -> ("Current"=w458:u32)  [unwired: 1 in, 2 out]
                    n206 = property class="DigNum (strict)"(reference=w457, error in=w447, "Value"=w458) -> (error out=w446:errorcluster)  [unwired: 1 out]
                  }
                }
                n207 = property class="CameraSettings"(reference=w412) -> ("ScanLineDelay"=w419:refnum<k24>, "ScanLineTime"=w418:refnum<k24>)  [unwired: 1 in, 2 out]
                n208 = property class="PmNumericParam`1[[System.UInt32"(reference=w419, error in=w420) -> (reference out=w422:refnum<k24>, error out=w421:errorcluster, "Available"=w423:bool)
                n209 = case shown="True" w423 {
                  tunnel: w430 -> [_ w441]
                  tunnel: w422 -> [_ w444]
                  tunnel: w421 -> [w439 w442]
                  tunnel: [w439 w443] -> w414
                  frame False {
                  }
                  frame True {
                    n210 = property class="PmNumericParam`1[[System.UInt32"(reference=w444) -> ("Current"=w440:u32)  [unwired: 1 in, 2 out]
                    n211 = property class="DigNum (strict)"(reference=w441, error in=w442, "Value"=w440) -> (error out=w443:errorcluster)  [unwired: 1 out]
                  }
                }
                n212 = property class="PmNumericParam`1[[System.Int64,"(reference=w418, error in=w414) -> (reference out=w416:refnum<k24>, error out=w413:errorcluster, "Available"=w417:bool)
                n213 = case shown="True" w417 {
                  tunnel: w416 -> [_ w438]
                  tunnel: w415 -> [_ w436]
                  tunnel: w413 -> [_ w435]
                  frame False {
                  }
                  frame True {
                    n214 = property class="PmNumericParam`1[[System.Int64,"(reference=w438, error in=w435) -> (error out=w434:errorcluster, "Current"=w437:i64)  [unwired: 1 out]
                    n215 = property class="DigNum (strict)"(reference=w436, error in=w434, "Value"=w437) -> ()  [unwired: 2 out]
                  }
                }
              }
            }
          }
          event "Exposure Time", "Trigger Out Behaviour": Value Change {
            n216 = local read "Camera Status"() -> (w459:bool)
            n217 = event-data() -> ()  [unwired: 1 in, 6 out]
            n218 = case shown="True" w459 {
              tunnel: w462 -> [w464 w468]
              tunnel: [w464 w465] -> w461
              frame False {
                n219 = One Button Dialog(message="Camera is not open") -> ()  [unwired: 1 in, 1 out]
              }
              frame True {
                w473 = 0 items=["Idle", "Capturing"] ("Status")
                n220 = property class="Camera"(reference=w468) -> (reference out=w466:refnum<k24>, "IsOpen"=w472:bool, "Status"=w474:i32)  [unwired: 1 in, 1 out]
                n221 = Equal?(x=w472, y=TRUE) -> (x = y?=w470:bool)
                n222 = Equal?(x=w474, y=w473) -> (x = y?=w469:bool)
                n223 = Equal?(x=w470, y=w469) -> (x = y?=w467:bool)
                n224 = case shown="True" w467 {
                  tunnel: w466 -> [w475 w492]
                  tunnel: [w475 w481] -> w465
                  frame False {
                  }
                  frame True {
                    n225 = property class="Camera"(reference=w492) -> (reference out=w481:refnum<k24>, "Settings"=w491:refnum<k24>)  [unwired: 1 in, 1 out]
                    n226 = control-ref of="Trigger Out Behaviour"() -> (w476:refnum<vi>)
                    n227 = control-ref of="Exp. out"() -> (w477:refnum<vi>)
                    n228 = property class="CameraSettings"(reference=w491) -> (reference out=w484:refnum<k24>, "ExposureTime"=w485:refnum<k24>, "ExposeOutMode"=w480:refnum<k24>)  [unwired: 1 in, 1 out]
                    n229 = property class="PmEnumParam"(reference=w480) -> (reference out=w478:refnum<k24>, "Available"=w479:bool)  [unwired: 1 in, 1 out]
                    n230 = property class="PmNumericParam`1[[System.UInt64"(reference=w485) -> (reference out=w488:refnum<k24>, "Max"=w490:u64, "Min"=w489:u64)  [unwired: 1 in, 1 out]
                    n231 = case shown="True" w479 {
                      tunnel: w478 -> [_ w502]
                      tunnel: w477 -> [_ w496]
                      tunnel: w476 -> [_ w493]
                      frame False {
                      }
                      frame True {
                        n232 = property class="CmbBox"(reference=w493) -> (reference out=w495:refnum<vi>, "Strings[]"=w503:string[])  [unwired: 1 in, 1 out]
                        n233 = property class="CmbBox"(reference=w495) -> ("Value"=w494:string)  [unwired: 1 in, 2 out]
                        n234 = while {
                          tunnel: w503 -> [w507] mode=indexing
                          tunnel: [w505] -> w500
                          tunnel: w494 -> [w504]
                          i -> [w505]
                          stop <- w506 stop-if-true
                          n235 = Equal?(x=w507, y=w504) -> (x = y?=w506:bool)
                        }
                        n236 = property class="PmEnumParam"(reference=w502) -> (reference out=w499:refnum<k24>, "Options"=w501:refnum<k24>)  [unwired: 1 in, 1 out]
                        n237 = invoke class="PmReadOnlyObservableCollection`" method="get_Item"(reference=w501, "index"=w500) -> ("get_Item"=w498:refnum<k24>)  [unwired: 2 in, 3 out]
                        n238 = property class="PmEnumItem"(reference=w498) -> ("Value"=w497:i32)  [unwired: 1 in, 2 out]
                        n239 = property class="PmEnumParam"(reference=w499, "Current"=w498) -> ()  [unwired: 1 in, 2 out]
                        n240 = property class="DigNum (strict)"(reference=w496, "Value"=w497) -> ()  [unwired: 1 in, 2 out]
                      }
                    }
                    n241 = local read "Exposure Time"() -> (w483:dbl)
                    n242 = In Range and Coerce(upper limit=w490, x=w483, lower limit=w489) -> (coerced(x)=w486:dbl)  [unwired: 1 out]
                    n243 = property class="CameraSettings"(reference=w484, "Exposure"=w486) -> ()  [unwired: 1 in, 2 out]
                    n244 = property class="PmNumericParam`1[[System.UInt64"(reference=w488, "Current"=w486) -> (reference out=w487:refnum<k24>)  [unwired: 1 in, 1 out]
                    n245 = property class="PmNumericParam`1[[System.UInt64"(reference=w487) -> ("Current"=w482:u64)  [unwired: 1 in, 2 out]
                    n246 = local write "Exposure Time"(w482) -> ()
                  }
                }
              }
            }
          }
          event "Live start": Value Change {
            n247 = event-data() -> ()  [unwired: 1 in, 6 out]
            n248 = case shown="True" "Live start" {
              tunnel: w510 -> [w512 w515]
              tunnel: [w512 w514] -> w509
              frame False {
              }
              frame True {
                n249 = local read "Camera Status"() -> (w513:bool)
                n250 = case shown="True" w513 {
                  tunnel: w515 -> [w516 w521]
                  tunnel: [w516 w519] -> w514
                  frame False {
                    n251 = One Button Dialog(message="Camera is not open") -> ()  [unwired: 1 in, 1 out]
                  }
                  frame True {
                    w526 = 0 items=["Idle", "Capturing"] ("Status")
                    n252 = property class="Camera"(reference=w521) -> (reference out=w520:refnum<k24>, "IsOpen"=w525:bool, "Status"=w527:i32)  [unwired: 1 in, 1 out]
                    n253 = Equal?(x=w525, y=TRUE) -> (x = y?=w523:bool)
                    n254 = Equal?(x=w527, y=w526) -> (x = y?=w522:bool)
                    n255 = Equal?(x=w523, y=w522) -> (x = y?=w518:bool)
                    n256 = case shown="True" w518 {
                      tunnel: w520 -> [w529 w531]
                      tunnel: [w529 w532] -> w519
                      frame False {
                        n257 = local write "Live"(FALSE ("Live 2")) -> ()
                      }
                      frame True {
                        n258 = flat-sequence {
                          tunnel: w531 -> [w537]
                          tunnel: [w534] -> w530
                          frame #0 {
                            n259 = property class="Camera"(reference=w537) -> (reference out=w534:refnum<k24>, "AcquisitionBuffer"=w536:refnum<k24>)  [unwired: 1 in, 1 out]
                            n260 = property class="AcqBuffer"(reference=w536, "BufferSize"=100) -> ()  [unwired: 1 in, 2 out]
                          }
                        }
                        n261 = local write "Live"(TRUE ("Live")) -> ()
                        n262 = invoke class="Camera" method="StartLive"(reference=w530) -> (reference out=w532:refnum<k24>)  [unwired: 2 in, 2 out]
                      }
                    }
                  }
                }
              }
            }
          }
          event "Live stop": Value Change {
            n263 = event-data() -> ()  [unwired: 1 in, 6 out]
            n264 = case shown="True" "Live stop" {
              tunnel: w539 -> [w541 w544]
              tunnel: [w541 w543] -> w538
              frame False {
              }
              frame True {
                n265 = local read "Camera Status"() -> (w542:bool)
                n266 = case shown="False" w542 {
                  tunnel: w544 -> [w546 w556]
                  tunnel: [w546 w553] -> w543
                  frame False {
                    n267 = One Button Dialog(message="Camera is not open") -> ()  [unwired: 1 in, 1 out]
                  }
                  frame True {
                    w551 = 1 items=["Idle", "Capturing"] ("Status")
                    n268 = property class="Camera"(reference=w556) -> (reference out=w554:refnum<k24>, "IsOpen"=w550:bool, "Status"=w552:i32)  [unwired: 1 in, 1 out]
                    n269 = Equal?(x=w552, y=w551) -> (x = y?=w547:bool)
                    n270 = Equal?(x=w550, y=TRUE) -> (x = y?=w548:bool)
                    n271 = Equal?(x=w548, y=w547) -> (x = y?=w555:bool)
                    n272 = case shown="True" w555 {
                      tunnel: w554 -> [w557 w560]
                      tunnel: [w557 w559] -> w553
                      frame False {
                      }
                      frame True {
                        n273 = invoke class="Camera" method="Stop"(reference=w560) -> (reference out=w559:refnum<k24>)  [unwired: 2 in, 2 out]
                        n274 = local write "Live"(FALSE ("Live 2")) -> ()
                      }
                    }
                  }
                }
              }
            }
          }
          event "Uninit": Value Change {
            n275 = event-data() -> ()  [unwired: 1 in, 6 out]
            n276 = case shown="True" "Uninit" {
              tunnel: w565 -> [w567 w571]
              tunnel: [w567 w570] -> w564
              tunnel: [FALSE ("Camera Status") w568] -> w562
              frame False {
              }
              frame True {
                n277 = local read "Camera Status"() -> (w569:bool)
                n278 = case shown="True" w569 {
                  tunnel: w571 -> [w573 w578]
                  tunnel: [w573 w577] -> w570
                  tunnel: [FALSE ("Camera Status") w576] -> w568
                  frame False {
                  }
                  frame True {
                    n279 = local read "Live"() -> (w574:bool)
                    n280 = Not(x=w574) -> (.not. x?=w575:bool)
                    n281 = case shown="True" w575 {
                      tunnel: w578 -> [w580 w583]
                      tunnel: [w580 w582] -> w577
                      tunnel: [FALSE ("Camera Status") w581] -> w576
                      frame False {
                      }
                      frame True {
                        n282 = flat-sequence {
                          tunnel: w583 -> [w586]
                          tunnel: [w585] -> w584
                          tunnel: [w589] -> w582
                          tunnel: w584 -> [w589]
                          tunnel: [TRUE ("Camera Status")] -> w581
                          frame #0 {
                            n283 = invoke class="Camera" method="Close"(reference=w586) -> (reference out=w585:refnum<k24>)  [unwired: 2 in, 2 out]
                          }
                          frame #1 {
                            n284 = local write "Camera Status"(FALSE ("Camera Status")) -> ()
                          }
                        }
                      }
                    }
                  }
                }
              }
            }
          }
        }
      }
    }
    frame #2 {
      n285 = invoke class="Library" method="Release"(reference=w591) -> (reference out=w592:refnum<k24>)  [unwired: 2 in, 2 out]
      n286 = Wait (ms)(milliseconds to wait=u32 100) -> ()  [unwired: 1 out]
      n287 = Close Reference(reference=w592) -> ()  [unwired: 1 in, 1 out]
    }
    frame #3 {
      n288 = invoke class="GC" method="Collect"() -> ()  [unwired: 3 in, 3 out]
    }
  }
  n289 = control-ref of="Exp. out"() -> (w1:refnum<vi>)
  n290 = property class="DigNum (strict)"(reference=w1, "Visible"=FALSE) -> ()  [unwired: 1 in, 2 out]
  n291 = control-ref of="Trigger Out Behaviour"() -> (w6:refnum<vi>)
  n292 = control-ref of="Exp. out"() -> (w4:refnum<vi>)
  n293 = property class="DigNum (strict)"(reference=w4, "Value"=0) -> ()  [unwired: 1 in, 2 out]
  n294 = property class="CmbBox"(reference=w6, "Value"="") -> ()  [unwired: 1 in, 2 out]
  n295 = local write "Camera Status"(FALSE ("Camera Status")) -> ()
  n296 = property on="Scan Width" class="DigNum (strict)"("DisabledEnum"=w9) -> ()  [unwired: 2 in, 2 out]
  n297 = property on="Scan Line Delay" class="DigNum (strict)"("DisabledEnum"=w9) -> ()  [unwired: 2 in, 2 out]
  n298 = control-ref of="Scan Line Delay"() -> (w12:refnum<vi>)
  n299 = control-ref of="Scan Width"() -> (w15:refnum<vi>)
  n300 = control-ref of="Scan Line Time"() -> (w11:refnum<vi>)
  n301 = control-ref of="Scan Direction"() -> (w18:refnum<vi>)
  n302 = control-ref of="Scan Mode"() -> (w21:refnum<vi>)
  n303 = property class="CmbBox"(reference=w21, "Value"="", "Strings[]"=string[] [] ("Strings []")) -> ()  [unwired: 1 in, 2 out]
  n304 = property class="DigNum (strict)"(reference=w12, "Value"=0.0) -> ()  [unwired: 1 in, 2 out]
  n305 = property class="CmbBox"(reference=w18, "Strings[]"=string[] [] ("Strings []"), "Value"="") -> ()  [unwired: 1 in, 2 out]
  n306 = property class="DigNum (strict)"(reference=w15, "Value"=0.0) -> ()  [unwired: 1 in, 2 out]
  n307 = property class="DigNum (strict)"(reference=w11, "Value"=0.0) -> ()  [unwired: 1 in, 2 out]
  n308 = local write "Scan Direction Reset"(FALSE ("Boolean")) -> ()
  "Boolean" <- FALSE ("Boolean")
